vi "CSM - Remove all CSM Bookmarks.vi"   [LabVIEW 2017]
doc: "### CSM - Remove All CSM Bookmarks.vi\n\nRemove all bookmarks in the CSM module."
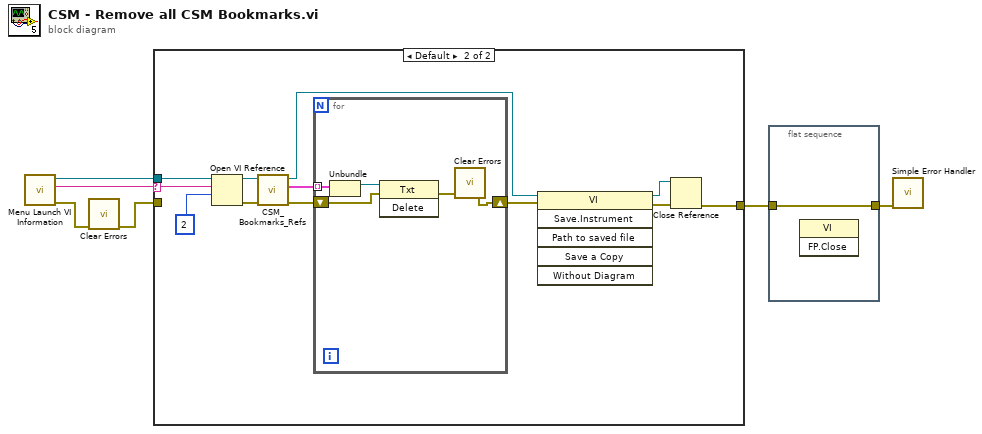
[diagram p0: block diagram]
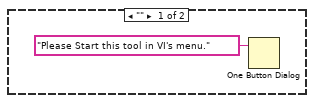
[diagram p2: hidden frame]
diagram:
  n1 = call <vilib>:"Menu Launch VI Information.vi"() -> ("error out"=w2:errorcluster, "Menu Launch:VI"=w5:string, "Menu Launch:App"=w6:refnum<vi>)  [unwired: 9 in]
  n2 = call <vilib>:"Clear Errors.vi"("error in (no error)"=w2) -> ("error out"=w1:errorcluster)  [unwired: 5 in, 1 out]
  n3 = case shown="Default" w5 {
    selector: w5 -> [_ w13]
    tunnel: w6 -> [_ w14]
    tunnel: [_ w8] -> w3
    tunnel: w1 -> [_ _]
    frame "" {
      n4 = One Button Dialog(message="Please Start this tool in VI's menu.") -> ()  [unwired: 1 in, 1 out]
    }
    frame Default {
      n5 = Open VI Reference(application reference (local)=w14, vi path=w13, options=2) -> (vi reference=w19:refnum<vi>, error out=w11:errorcluster)  [unwired: 3 in]
      n6 = call "CSM_Bookmarks_Refs.vi"("error in (no error)"=w11, "VIRef"=w19) -> ("error out"=w17:errorcluster, "Array"=w18:cluster{refnum<vi>, "Text":string}[], "Reference Out"=w15:refnum<vi>)  [unwired: 7 in]
      n7 = for {
        tunnel: w18 -> [w24] mode=indexing
        shift-right: [w20] -> w16
        shift-left: w17 -> [w22]
        n8 = Unbundle(w24) -> (w23:refnum<vi>)  [unwired: 1 out]
        n9 = invoke class="Txt" method="Delete"(reference=w23, error in=w22) -> (error out=w21:errorcluster)  [unwired: 1 in, 2 out]
        n10 = call <vilib>:"Clear Errors.vi"("error in (no error)"=w21) -> ("error out"=w20:errorcluster)  [unwired: 5 in, 1 out]
      }
      n11 = invoke class="VI" method="Save.Instrument"(reference=w15, error in=w16) -> (reference out=w10:refnum<vi>, error out=w9:errorcluster)  [unwired: 4 in, 4 out]
      n12 = Close Reference(reference=w10, error in (no error)=w9) -> (error out=w8:errorcluster)
    }
  }
  n13 = flat-sequence {
    tunnel: [w25] -> w4
    tunnel: w3 -> [w25]
    frame #0 {
      n14 = invoke class="VI" method="FP.Close"() -> ()  [unwired: 3 in, 3 out]
    }
  }
  n15 = call <vilib>:"Simple Error Handler.vi"("error in (no error)"=w4) -> ()  [unwired: 4 in, 5 out]
